vi "G-DataType-To-Go.vi"(8 "error in (no error)":errorcluster, 11 "CMD":variant) -> (0 "error out":errorcluster, 3 "result string":string)   [LabVIEW 2020, in "Generate-Go-CMD.lvlib"]
uses:
  Generate-Go-CMD.lvlib
  <vilib>/Utility/Data Type/NI_Data Type.lvlib
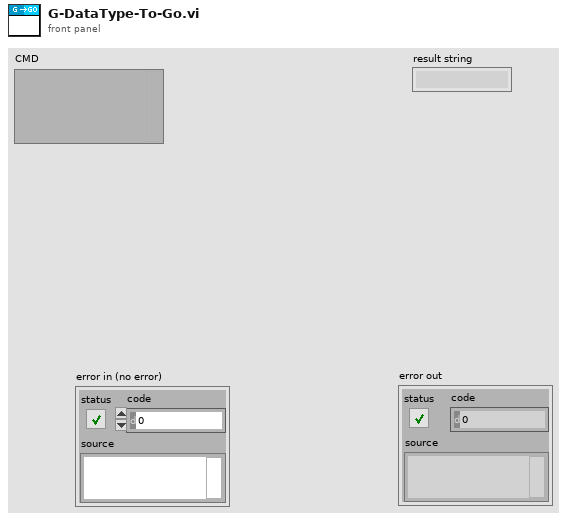
[diagram p1: front panel]
types:
  T1 = typedef "NI_Data Type.lvlib/Data Type.ctl" = enum8{"Invalid Type", "Void", "I8", "I16", "I32", "I64", "U8", "U16", "U32", "U64", "Single Float", "Double Float", "Extended Float", "Single Complex", "Double Complex", "Extended Complex", "Enum U8", "Enum U16", "Enum U32", "Enum U64", "Single Float With Unit", "Double Float With Unit", "Extended Float With Unit", "Single Complex with Unit", "Double Complex with Unit", "Extended Complex with Unit", "Boolean", "String", "Path", "Picture", "Tag", "Array", "Cluster", "Variant", "LV Variant", "Waveform", "Timestamp", "Digital Waveform", "Digital Data", "ExpressData", "Refnum", "External Data", "VI", "Poly VI", "LabVIEW Class Instance", "Fixed Point", "Set Collection", "Map Collection"}
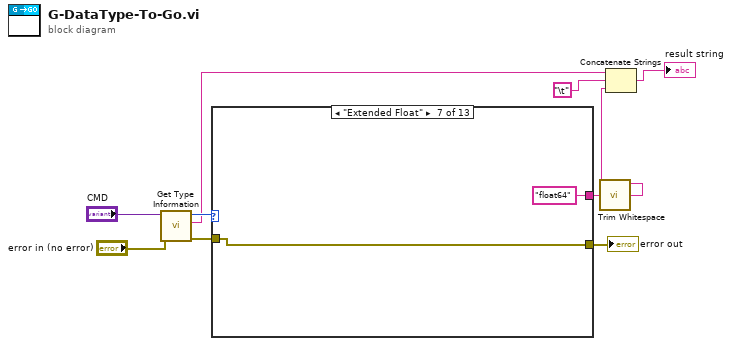
[diagram p0: block diagram]
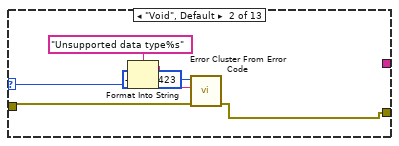
[diagram p3: hidden frame]
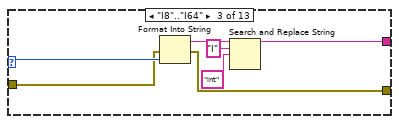
[diagram p4: hidden frame]
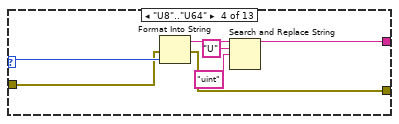
[diagram p5: hidden frame]
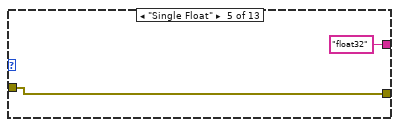
[diagram p6: hidden frame]
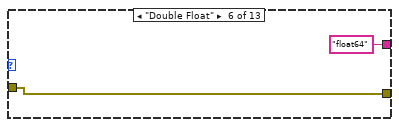
[diagram p7: hidden frame]
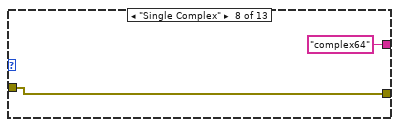
[diagram p8: hidden frame]
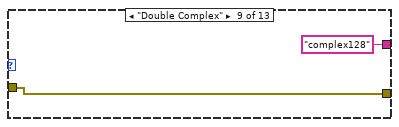
[diagram p9: hidden frame]
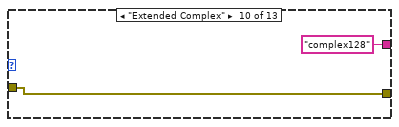
[diagram p10: hidden frame]
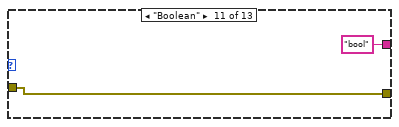
[diagram p11: hidden frame]
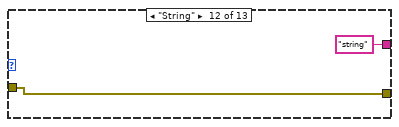
[diagram p12: hidden frame]
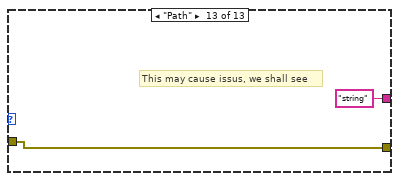
[diagram p13: hidden frame]
diagram:
  n1 = call <vilib>:"Get Type Information.vi"("error in (no error)"="error in (no error)", "variant"="CMD") -> ("error out"=w6:errorcluster, "name"=w2:string, "type"=w8:T1)  [unwired: 5 in, 2 out]
  n2 = case shown="\"Extended Float\"" w8 {
    selector: w8 -> [_ w16 w24 w31 _ _ _ _ _ _ _ _ _]
    tunnel: [_ _ w20 w27 "float32" ("result string") "float64" ("result string") "float64" ("result string") "complex64" ("result string") "complex128" ("result string") "complex128" ("result string") "bool" ("result string") "string" ("result string") "string" ("result string")] -> w7
    tunnel: w6 -> [w11 w17 w19 w26 w32 w34 w36 w38 w40 w42 w44 w46 w48]
    tunnel: [w11 w13 w18 w25 w32 w34 w36 w38 w40 w42 w44 w46 w48] -> w5
    frame "Invalid Type" {
    }
    frame "Void", Default {
      n3 = Format Into String(format string="Unsupported data type%s", w16) -> (resulting string=w15:string)  [unwired: 2 in, 1 out]
      n4 = call <vilib>:"Error Cluster From Error Code.vi"("error in (no error)"=w17, "error message (\"\")"=w15, "error code (0)"=-98328423) -> ("error out"=w13:errorcluster)  [unwired: 6 in]
    }
    frame "I8".."I64" {
      n5 = Format Into String(error in=w19, w24) -> (resulting string=w23:string, error out=w18:errorcluster)  [unwired: 2 in]
      n6 = Search and Replace String(input string=w23, search string="I", replace string="int" ("search string")) -> (result string=w20:string)  [unwired: 5 in, 3 out]
    }
    frame "U8".."U64" {
      n7 = Format Into String(error in=w26, w31) -> (resulting string=w30:string, error out=w25:errorcluster)  [unwired: 2 in]
      n8 = Search and Replace String(input string=w30, search string="U", replace string="uint" ("search string")) -> (result string=w27:string)  [unwired: 5 in, 3 out]
    }
    frame "Single Float" {
    }
    frame "Double Float" {
    }
    frame "Extended Float" {
    }
    frame "Single Complex" {
    }
    frame "Double Complex" {
    }
    frame "Extended Complex" {
    }
    frame "Boolean" {
    }
    frame "String" {
    }
    frame "Path" {
      # "This may cause issus, we shall see"
    }
  }
  "error out" <- w5
  n9 = call <vilib>:"Trim Whitespace.vi"("string"=w7) -> ("trimmed string"=w4:string)  [unwired: 1 in]
  n10 = Concatenate Strings(w2, "\t", w4) -> (→"result string":string)
